vi "PWMLimiter.vi"(10 "Cluster":cluster{"PWM_demand":i32, "V1":bool}={"PWM_demand"=0, "V1"=TRUE}) -> (1 "Boolean":bool, 2 "PWM":i32)   [LabVIEW 2015]
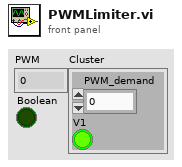
[diagram p1: front panel]
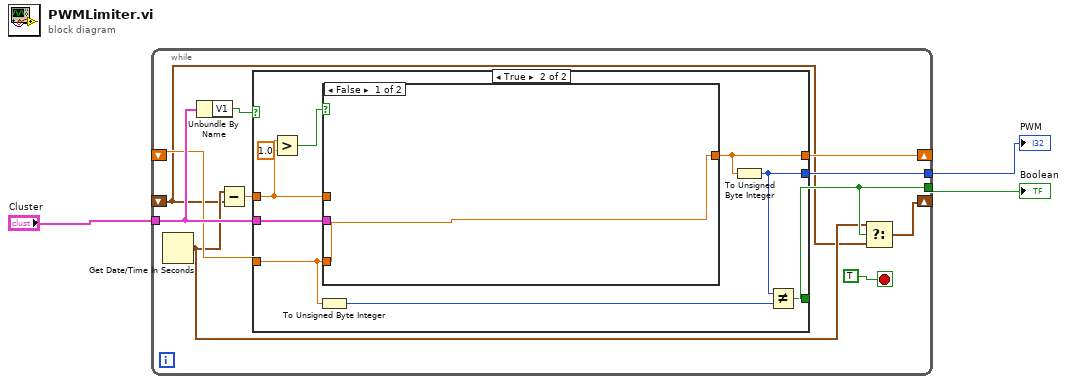
[diagram p0: block diagram]
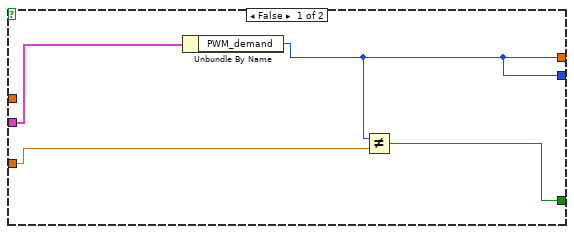
[diagram p2: hidden frame]
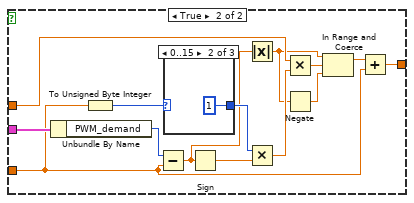
[diagram p3: hidden frame]
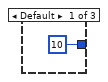
[diagram p4: hidden frame]
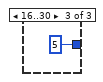
[diagram p5: hidden frame]
diagram:
  n1 = while {
    tunnel: "Cluster" -> [w14]
    tunnel: [w7] -> w2
    shift-right: [w4] -> _
    shift-left: _ -> [w5]
    shift-right: [w12] -> _
    shift-left: _ -> [w11]
    tunnel: [w10] -> w1
    stop <- TRUE stop-if-true
    n2 = Get Date/Time In Seconds() -> (seconds since 1Jan1904=w6:timestamp)
    n3 = Unbundle By Name(w14) -> ("V1"=w8:bool)
    n4 = Subtract(x=w6, y=w5) -> (x-y=w9:dbl)
    n5 = case shown="True" w8 {
      tunnel: w14 -> [w18 w27]
      tunnel: [w15 w26] -> w7
      tunnel: [w17 w24] -> w12
      tunnel: w11 -> [w16 w23]
      tunnel: [w17 w22] -> w10
      tunnel: w9 -> [_ w21]
      frame False {
        n6 = Unbundle By Name(w18) -> ("PWM_demand"=w17:i32)
        n7 = Not Equal?(x=w17, y=w16) -> (x != y?=w15:bool)
      }
      frame True {
        n8 = Greater?(x=w21, y=1.0) -> (0:w19:bool)
        n9 = To Unsigned Byte Integer(number=w23) -> (unsigned 8bit integer=w25:u8)
        n10 = case shown="False" w19 {
          tunnel: w27 -> [_ w42]
          tunnel: [w28 w36] -> w24
          tunnel: w23 -> [w28 w35]
          tunnel: w21 -> [_ w37]
          frame False {
          }
          frame True {
            n11 = Unbundle By Name(w42) -> ("PWM_demand"=w41:i32)
            n12 = To Unsigned Byte Integer(number=w35) -> (unsigned 8bit integer=w34:u8)
            n13 = Subtract(x=w41, y=w35) -> (x-y=w31:dbl)
            n14 = case shown="0..15" w34 {
              tunnel: [10 1 5] -> w40
              frame Default {
              }
              frame 0..15 {
              }
              frame 16..30 {
              }
            }
            n15 = Sign(1:w31) -> (0:w39:dbl)
            n16 = Absolute Value(x=w31) -> (abs(x)=w30:dbl)
            n17 = Multiply(x=w40, y=w39) -> (x*y=w38:dbl)
            n18 = Multiply(x=w37, y=w38) -> (x*y=w33:dbl)
            n19 = Negate(x=w30) -> (-x=w29:dbl)
            n20 = In Range and Coerce(upper limit=w30, x=w33, lower limit=w29) -> (coerced(x)=w32:dbl)  [unwired: 1 out]
            n21 = Add(x=w32, y=w35) -> (x+y=w36:dbl)
          }
        }
        n22 = To Unsigned Byte Integer(number=w24) -> (unsigned 8bit integer=w22:u8)
        n23 = Not Equal?(x=w22, y=w25) -> (x != y?=w26:bool)
      }
    }
    n24 = Select(t=w6, s=w7, f=w5) -> (s? t:f=w4:timestamp)
  }
  "PWM" <- w1
  "Boolean" <- w2
